vi "Make Caption.vi"(6 "Mode":enum16{"Libraries", "Variables"}(ring), 8 "size(s)":i32) -> (0 "Caption":string)   [LabVIEW 2014]
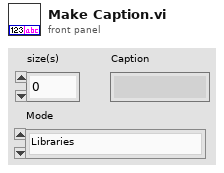
[diagram p1: front panel]
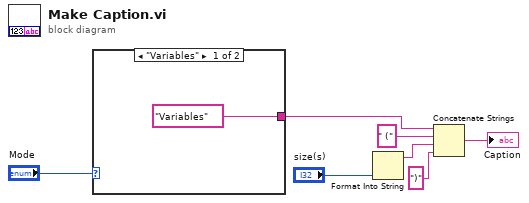
[diagram p0: block diagram]
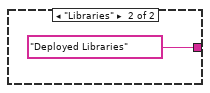
[diagram p2: hidden frame]
diagram:
  n1 = case shown="\"Variables\"" "Mode" {
    tunnel: ["Variables" "Deployed Libraries"] -> w3
    frame "Variables" {
    }
    frame "Libraries" {
    }
  }
  n2 = Format Into String("size(s)") -> (resulting string=w5:string)  [unwired: 3 in, 1 out]
  n3 = Concatenate Strings(w3, " (" ("string"), w5, ")" ("string")) -> (→"Caption":string)
